vi "Copy Class.vi"(11 "Actor Script Strategy in":refnum<class "Actor Script Strategy.lvclass">) -> (0 "error out":errorcluster, 3 "Actor Script Strategy out":refnum<class "Actor Script Strategy.lvclass">)   [LabVIEW 2021, in "_Create From Template.lvlib" / "Script Strategy.lvlib" / "Actor Script Strategy.lvclass"]
uses:
  Actor Script Strategy.lvclass
  Actor Script Strategy.lvclass/Actor Script Strategy.ctl
  _Create From Template.lvlib
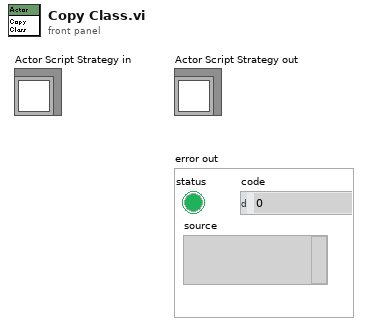
[diagram p1: front panel]
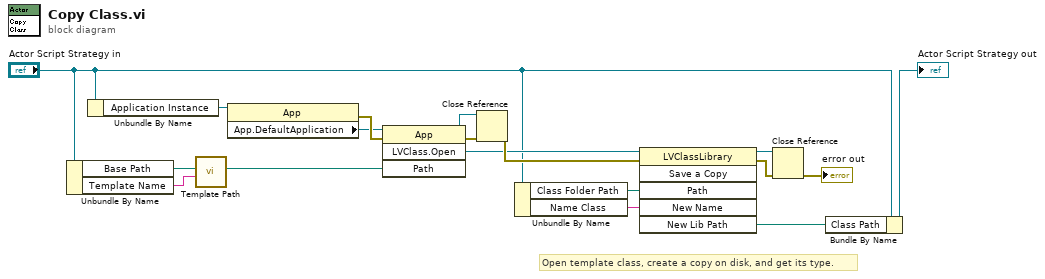
[diagram p0: block diagram]
diagram:
  # "Open template class, create a copy on disk, and get its type."
  n1 = Unbundle By Name("Actor Script Strategy in") -> ("Base Path"=w2:path, "Template Name"=w1:string)
  n2 = Unbundle By Name("Actor Script Strategy in") -> ("Application Instance"=w10:refnum<vi>)
  n3 = call "Template Path.vi"("Template Name"=w1, "Base Path"=w2) -> ("Template Path"=w4:path)  [unwired: 9 in]
  n4 = property class="App"(reference=w10) -> (error out=w17:errorcluster, "App.DefaultApplication"=w12:refnum<vi>)  [unwired: 1 in, 1 out]
  n5 = invoke class="App" method="LVClass.Open"(reference=w12, error in=w17, "Path"=w4) -> (reference out=w11:refnum<vi>, error out=w18:errorcluster, "LVClass.Open"=w14:refnum<vi>)  [unwired: 1 in, 1 out]
  n6 = Close Reference(reference=w11, error in (no error)=w18) -> (error out=w15:errorcluster)
  n7 = Unbundle By Name("Actor Script Strategy in") -> ("Class Folder Path"=w8:path, "Name Class"=w9:string)
  n8 = invoke class="LVClassLibrary" method="Save a Copy"(reference=w14, error in=w15, "Path"=w8, "New Name"=w9) -> (reference out=w13:refnum<vi>, error out=w5:errorcluster, "New Lib Path"=w6:path)  [unwired: 2 in, 3 out]
  n9 = Close Reference(reference=w13, error in (no error)=w5) -> (error out=→"error out":errorcluster)
  n10 = Bundle By Name(cluster="Actor Script Strategy in", "Class Path"=w6) -> (→"Actor Script Strategy out":refnum<class "Actor Script Strategy.lvclass">)
